vi "kvCanObjBufDisable.vi"(2 "error in (no error)":errorcluster, 3 "Output Handle":i32, 4 "Channel Handle (input only)":i32) -> (0 "error out":errorcluster, 1 "Channel Handle (output only)":i32)   [LabVIEW 2022 SP3]
doc: "Stops the specified object buffers transmission activities."
uses:
  canlib32.dll
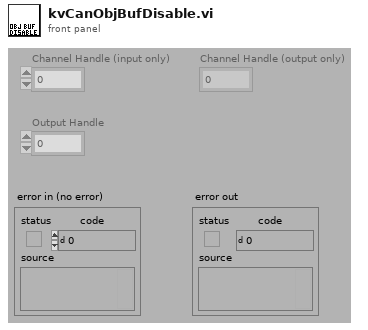
[diagram p1: front panel]
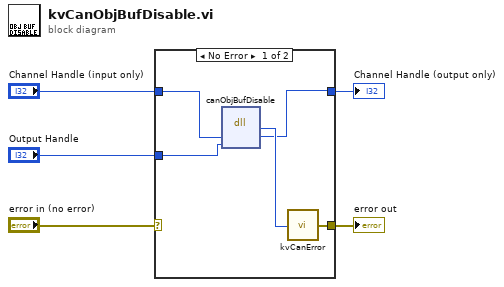
[diagram p0: block diagram]
diagram:
  n1 = case shown="No Error" "error in (no error)" {
    selector: "error in (no error)" -> [_ w11]
    tunnel: "Channel Handle (input only)" -> [w8 w12]
    tunnel: [w6 w12] -> w3
    tunnel: [w10 w11] -> w2
    tunnel: "Output Handle" -> [w7 _]
    frame No Error {
      n2 = dll-call lib="canlib32.dll" fn="canObjBufDisable"("channelHandle"=w8, "objectHandle"=w7) -> (w9:i32, "channelHandle"=w6:i32)  [unwired: 4 in, 2 out]
      n3 = call "kvCanError.vi"("error code"=w9) -> ("error out"=w10:errorcluster)
    }
    frame Error {
    }
  }
  "error out" <- w2
  "Channel Handle (output only)" <- w3
